vi "Read 01-00-9213.vi"(8 "error in":errorcluster) -> (0 "error out":errorcluster, 3 "01-00-9213":dbl[](array[numeric]))   [LabVIEW 2018, in "Inputs.lvlib"]
uses:
  Inputs.lvlib
  <vilib>/ptbypt/Probability & Statistics.llb/Mean PtByPt.vi
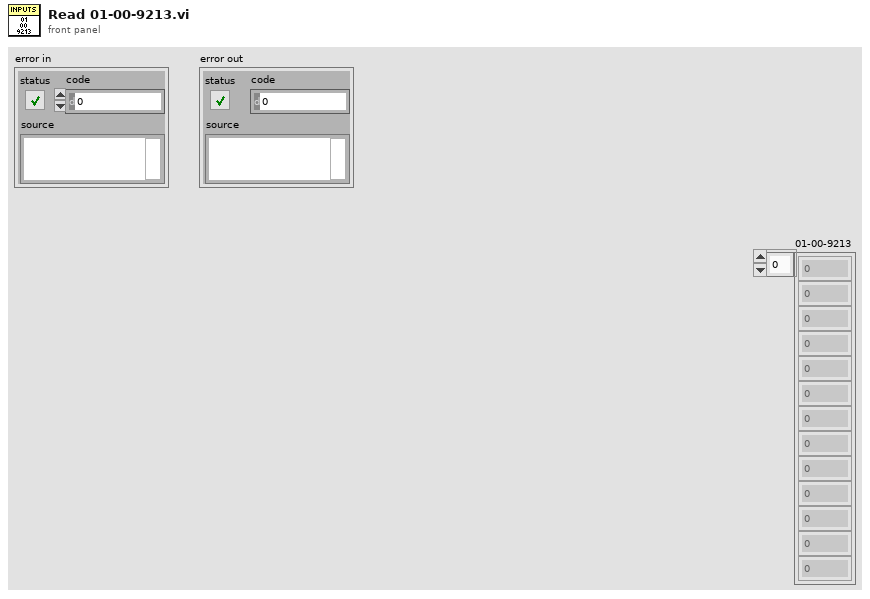
[diagram p1: front panel]
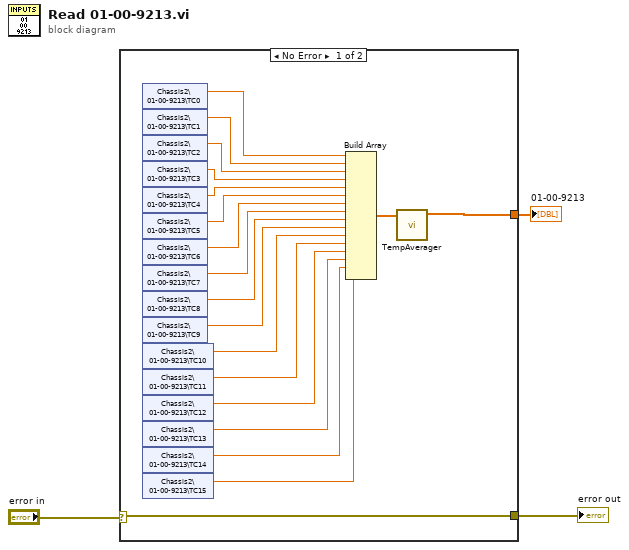
[diagram p0: block diagram]
diagram:
  n1 = case shown="No Error" "error in" {
    selector: "error in" -> [w22 w23]
    tunnel: [w22 w23] -> w3
    tunnel: [w21 _] -> w1
    frame No Error {
      n2 = shared-variable "Chassis2\\01-00-9213\\TC0"() -> (w20:dbl)  [unwired: 1 in, 1 out]
      n3 = shared-variable "Chassis2\\01-00-9213\\TC1"() -> (w19:dbl)  [unwired: 1 in, 1 out]
      n4 = shared-variable "Chassis2\\01-00-9213\\TC2"() -> (w18:dbl)  [unwired: 1 in, 1 out]
      n5 = shared-variable "Chassis2\\01-00-9213\\TC3"() -> (w17:dbl)  [unwired: 1 in, 1 out]
      n6 = shared-variable "Chassis2\\01-00-9213\\TC4"() -> (w16:dbl)  [unwired: 1 in, 1 out]
      n7 = shared-variable "Chassis2\\01-00-9213\\TC5"() -> (w15:dbl)  [unwired: 1 in, 1 out]
      n8 = shared-variable "Chassis2\\01-00-9213\\TC6"() -> (w14:dbl)  [unwired: 1 in, 1 out]
      n9 = shared-variable "Chassis2\\01-00-9213\\TC7"() -> (w13:dbl)  [unwired: 1 in, 1 out]
      n10 = shared-variable "Chassis2\\01-00-9213\\TC8"() -> (w12:dbl)  [unwired: 1 in, 1 out]
      n11 = shared-variable "Chassis2\\01-00-9213\\TC9"() -> (w11:dbl)  [unwired: 1 in, 1 out]
      n12 = shared-variable "Chassis2\\01-00-9213\\TC10"() -> (w10:dbl)  [unwired: 1 in, 1 out]
      n13 = shared-variable "Chassis2\\01-00-9213\\TC11"() -> (w9:dbl)  [unwired: 1 in, 1 out]
      n14 = shared-variable "Chassis2\\01-00-9213\\TC12"() -> (w8:dbl)  [unwired: 1 in, 1 out]
      n15 = shared-variable "Chassis2\\01-00-9213\\TC13"() -> (w7:dbl)  [unwired: 1 in, 1 out]
      n16 = shared-variable "Chassis2\\01-00-9213\\TC14"() -> (w6:dbl)  [unwired: 1 in, 1 out]
      n17 = shared-variable "Chassis2\\01-00-9213\\TC15"() -> (w5:dbl)  [unwired: 1 in, 1 out]
      n18 = Build Array(w20, w19, w18, w17, w16, w15, w14, w13, w12, w11, w10, w9, w8, w7, w6, w5) -> (w4:dbl[])
      n19 = call "TempAverager.vi"("Array in"=w4) -> ("Array out"=w21:dbl[])  [unwired: 10 in]
    }
    frame Error {
    }
  }
  "error out" <- w3
  "01-00-9213" <- w1
